vi "Update-status.vi"(6 "Status":T1, 8 "error in (no error)":errorcluster, 11 "Object ref in":T2) -> (0 "error out":errorcluster, 3 "Object ref out":T2)   [LabVIEW 2013, in "PowderDeposition.lvlib" / "PD-Main.lvclass"]
uses:
  PD-Main.lvclass
  Object-reference.ctl
  Client-status.ctl
  PD-Main.lvclass/PD-Main.ctl
  Read Client status.vi
  Write Status.vi
  Read Client.vi
  Communication/Sources/PD-Client.lvclass
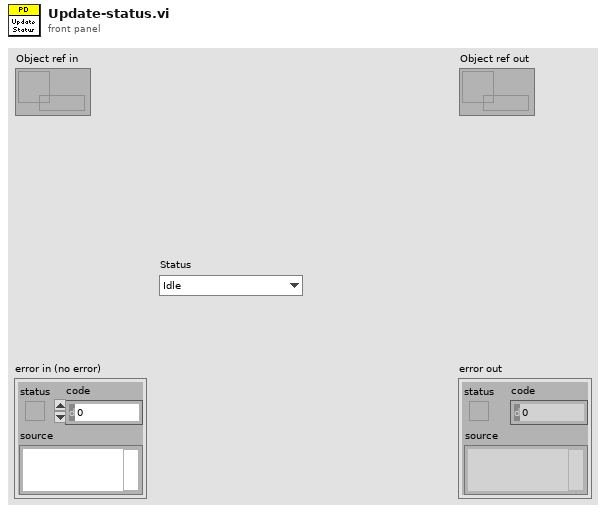
[diagram p1: front panel]
types:
  T1 = typedef "PowderDeposition.lvlib/PD-Main.lvclass/Client-status.ctl" = enum16{"Idle", "Initialized", "Configured", "Activated", "Started", "Paused", "Stopped", "Reset", "Error", "Exited"}
  T2 = typedef "PowderDeposition.lvlib/PD-Main.lvclass/Object-reference.ctl" = refnum<data-value>
  T3 = typedef "PowderDeposition.lvlib/PD-Client.lvclass/Object-reference.ctl" = refnum<data-value>
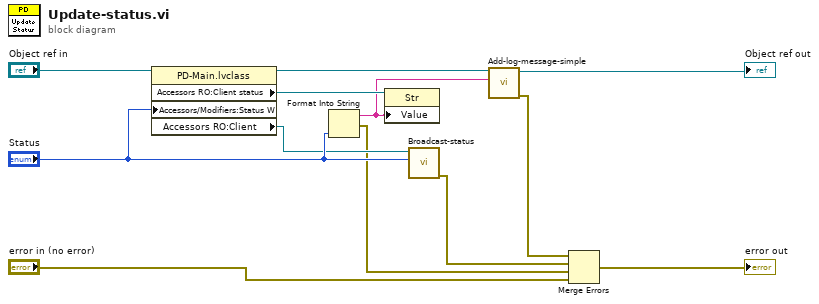
[diagram p0: block diagram]
diagram:
  n1 = property class="PD-Main.lvclass"(reference="Object ref in", "Accessors/Modifiers:Status W"="Status") -> (reference out=w4:T2, "Accessors RO:Client status"=w9:refnum<vi>, "Accessors RO:Client"=w7:T3)  [unwired: 1 in, 1 out]
  n2 = Format Into String("Status") -> (resulting string=w2:string, error out=w6:errorcluster)  [unwired: 3 in]
  n3 = property class="Str"(reference=w9, "Value"=w2) -> ()  [unwired: 1 in, 2 out]
  n4 = call "Broadcast-status.vi"("Status"="Status", "Client in"=w7) -> ("error out"=w12:errorcluster)  [unwired: 8 in, 1 out]
  n5 = call "Add-log-message-simple.vi"("Message"=w2, "UI in"=w4) -> ("error out"=w1:errorcluster, "UI out"=→"Object ref out":T2)  [unwired: 8 in]
  n6 = Merge Errors(w1, w12, w6, "error in (no error)") -> (→"error out":errorcluster)
